vi "delete subVI on the other end of this wire.vi"(8 "error in":errorcluster, 10 "wire":refnum<vi>, 11 "source term":refnum<vi>) -> (0 "error out":errorcluster, 3 "connected terminals":refnum<vi>[](array[refnum]))   [LabVIEW 2014, in "SequencerActionScript.lvclass"]
doc: "NI Tag Bus Module Framework 1.0.2.36\nNI Systems Engineering"
uses:
  SequencerActionScript.lvclass
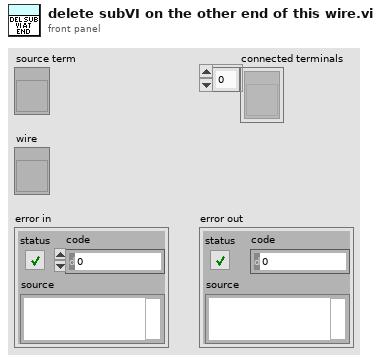
[diagram p1: front panel]
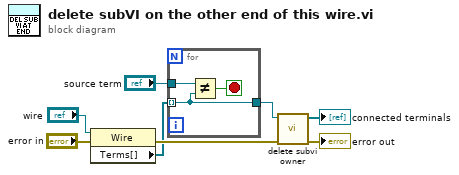
[diagram p0: block diagram]
diagram:
  n1 = property class="Wire"(reference="wire", error in="error in") -> (error out=w6:errorcluster, "Terms[]"=w3:refnum<vi>[])  [unwired: 1 out]
  n2 = for {
    tunnel: w3 -> [w9] mode=indexing
    tunnel: "source term" -> [w11]
    tunnel: [w9] -> w5
    stop <- w10 stop-if-true
    n3 = Not Equal?(x=w11, y=w9) -> (x != y?=w10:bool)
  }
  n4 = call "delete subvi owner.vi"("error in"=w6, "terminal in"=w5) -> ("error out"=→"error out":errorcluster, "other terminals"=→"connected terminals":refnum<vi>[])  [unwired: 8 in]
